vi "Write isLeftClick.vi"(8 "error in (no error)":errorcluster, 10 "isLeftClick?":bool, 11 "ModeCol in":refnum<class "ModeCol.lvclass">) -> (0 "error out":errorcluster, 3 "ModeCol out":refnum<class "ModeCol.lvclass">)   [LabVIEW 2013, in "ModeCol.lvclass"]
uses:
  ModeCol.lvclass
  ModeCol.lvclass/ModeCol.ctl
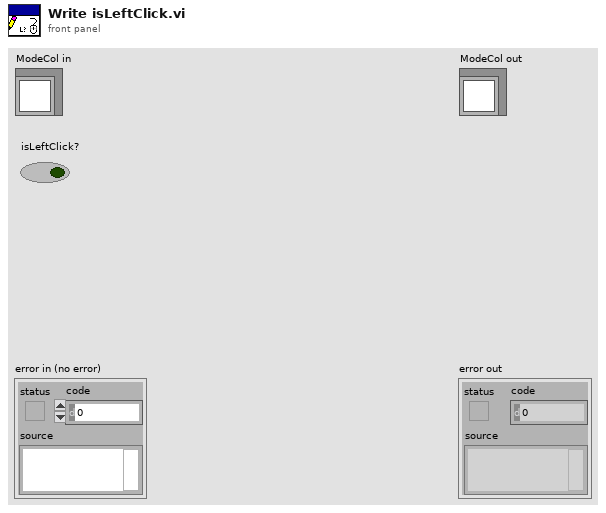
[diagram p1: front panel]
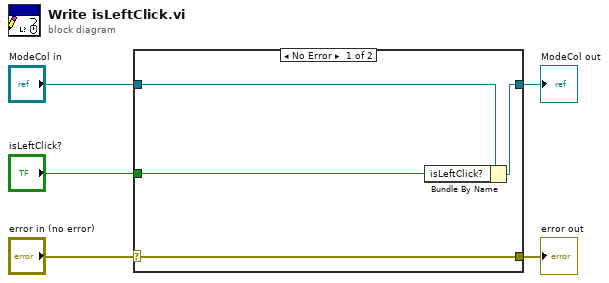
[diagram p0: block diagram]
diagram:
  n1 = case shown="No Error" "error in (no error)" {
    selector: "error in (no error)" -> [w9 w10]
    tunnel: [w9 w10] -> w4
    tunnel: [w7 w11] -> w2
    tunnel: "ModeCol in" -> [w8 w11]
    tunnel: "isLeftClick?" -> [w6 _]
    frame No Error {
      n2 = Bundle By Name(cluster=w8, "isLeftClick?"=w6) -> (w7:refnum<class "ModeCol.lvclass">)
    }
    frame Error {
    }
  }
  "error out" <- w4
  "ModeCol out" <- w2
